vi "Write connection information.vi"(8 "error in (no error)":errorcluster, 10 "connection information":string, 11 "BaseMeasurement in":refnum<class "BaseMeasurement.lvclass">) -> (0 "error out":errorcluster, 3 "BaseMeasurement out":refnum<class "BaseMeasurement.lvclass">)   [LabVIEW 2013, in "BaseMeasurement.lvclass"]
doc: "This accessor can be used to set the file path for the data file."
uses:
  BaseMeasurement.lvclass
  BaseMeasurement.lvclass/BaseMeasurement.ctl
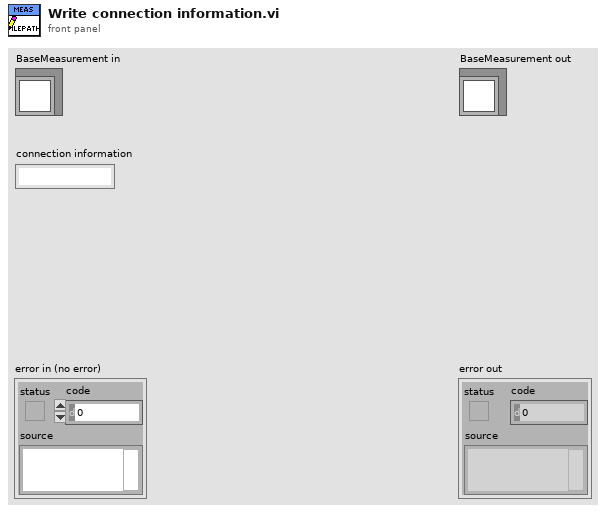
[diagram p1: front panel]
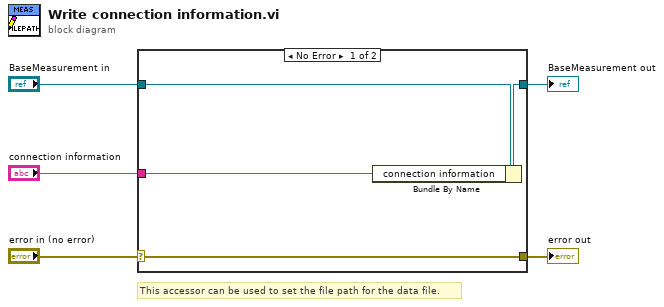
[diagram p0: block diagram]
diagram:
  # "This accessor can be used to set the file path for the data file."
  n1 = case shown="No Error" "error in (no error)" {
    selector: "error in (no error)" -> [w9 w10]
    tunnel: [w9 w10] -> w4
    tunnel: [w7 w11] -> w2
    tunnel: "BaseMeasurement in" -> [w8 w11]
    tunnel: "connection information" -> [w6 _]
    frame No Error {
      n2 = Bundle By Name(cluster=w8, "connection information"=w6) -> (w7:refnum<class "BaseMeasurement.lvclass">)
    }
    frame Error {
    }
  }
  "error out" <- w4
  "BaseMeasurement out" <- w2
